vi "LabVIEW Time Stampt to Time Stamp 64.vi"(8 "Error In":errorcluster, 11 "LabVIEW Time Stamp":timestamp) -> (0 "Error Out":errorcluster, 3 "Time Stamp 64":T1)   [LabVIEW 2019, in "SNTP.lvlib"]
uses:
  SNTP.lvlib
  Public/Controls/Time Stamp 64.ctl
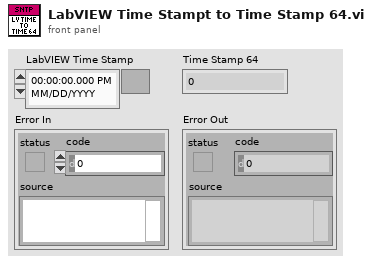
[diagram p1: front panel]
types:
  T1 = typedef "SNTP.lvlib/Time Stamp 64.ctl" = fxp<+,64,32>
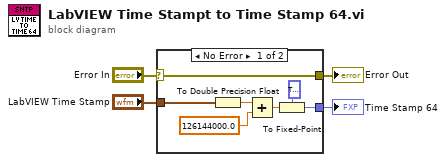
[diagram p0: block diagram]
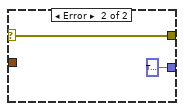
[diagram p2: hidden frame]
diagram:
  n1 = case shown="No Error" "Error In" {
    selector: "Error In" -> [w10 w13]
    tunnel: [w10 w13] -> w3
    tunnel: "LabVIEW Time Stamp" -> [w9 _]
    tunnel: [w7 T1 0.0 ("Time Stamp 64")] -> w1
    frame No Error {
      n2 = To Double Precision Float(number=w9) -> (double precision float=w11:dbl)
      n3 = Add(x=w11, y=126144000.0) -> (x+y=w8:dbl)
      n4 = To Fixed-Point(fixed-point type=T1 0.0 ("Time Stamp 64"), number=w8) -> (fixed-point=w7:T1)
    }
    frame Error {
    }
  }
  "Error Out" <- w3
  "Time Stamp 64" <- w1
